vi "Get Desired Size.vi"(8 "error in (no error)":errorcluster, 11 "Team Config Panel in":refnum<class "Team Config Panel.lvclass">) -> (0 "error out":errorcluster, 2 "Desired Size":T1, 3 "Team Config Panel out":refnum<class "Team Config Panel.lvclass">)   [LabVIEW 2020, in "SB App.lvlib" / "Team Config Panel.lvclass"]
uses:
  Team Config Panel.lvclass
  <vilib>/IlluminatedG/IG OOPanel/OOPanel/ArrayPanel/Desired Size.ctl
  Team Config Panel.lvclass/Team Config Panel.ctl
  <vilib>/IlluminatedG/IG OOPanel/OOPanel/OOPanel.lvlib
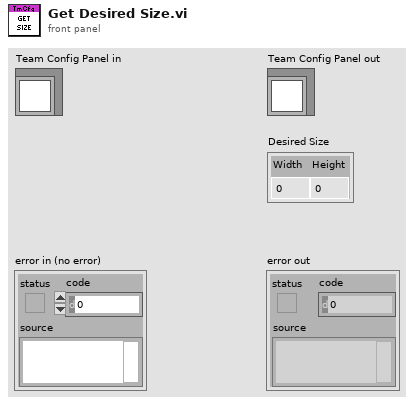
[diagram p1: front panel]
types:
  T1 = typedef "OOPanel.lvlib/Desired Size.ctl" = cluster{"Width":u32, "Height":u32}
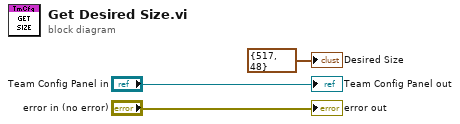
[diagram p0: block diagram]
diagram:
  "error out" <- "error in (no error)"
  "Team Config Panel out" <- "Team Config Panel in"
  "Desired Size" <- T1 {"Width"=517, "Height"=48} ("Desired Size")
